vi "setUp.vi"(8 "error in":errorcluster, 11 "reference in":refnum<class "Single Board Loopback.lvclass">) -> (0 "error out":errorcluster, 3 "reference out":refnum<class "Single Board Loopback.lvclass">)   [LabVIEW 2020, in "Single Board Loopback.lvclass"]
doc: "setUp runs prior to the test method during test execution. Use this method to initialize any object data required by your tests."
uses:
  Single Board Loopback.lvclass
  C:/Program Files (x86)/National Instruments/LabVIEW 2020/vi.lib/addons/_JKI Toolkits/VI Tester/TestCase.llb/TestCase.lvclass
  <vilib>/addons/_JKI Toolkits/VI Tester/TestCase.llb/TestCase.lvclass
  C:/Users/nitest/Desktop/Git 2020/niveristand-custom-device-testing-tools/VeriStandTestCase/VeriStandTestCase.lvclass
  C:/Users/nitest/Desktop/Git 2020/niveristand-aim-arinc429-custom-device/Source/Custom Device Support/Tests/System/Single Board Loopback/Single Board Loopback.lvclass
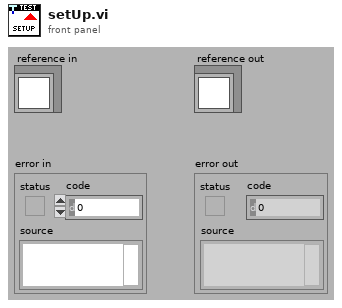
[diagram p1: front panel]
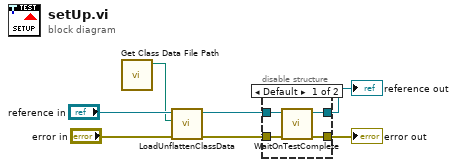
[diagram p0: block diagram]
diagram:
  n1 = call "Get Class Data File Path.vi"() -> ("Class Data File Path"=w3:path)  [unwired: 11 in]
  n2 = call-dynamic "LoadUnflattenClassData.vi"("error in"="error in", "Class Data File Path"=w3, "VeriStandTestCase in"="reference in") -> ("error out"=w2:errorcluster, "VeriStandTestCase out"=w1:refnum<class "Single Board Loopback.lvclass">)  [unwired: 7 in]
  n3 = disable-structure shown="Default" {
    disable-tunnel: w2 -> [w11 w12]
    disable-tunnel: [w10 w12] -> w7
    disable-tunnel: [w9 w13] -> w6
    disable-tunnel: w1 -> [w8 w13]
    frame condition #0 (active) {
      n4 = call <vilib>:"WaitOnTestComplete.vi"("error in (no error)"=w11, "TestCase in"=w8) -> ("error out"=w10:errorcluster, "TestCase out"=w9:refnum<class "Single Board Loopback.lvclass">)  [unwired: 8 in]
    }
    frame condition #1 {
    }
  }
  "error out" <- w7
  "reference out" <- w6
